vi "lbvproject.vi"() -> ()   [LabVIEW 2023]
uses:
  <vilib>/measure/mamon.llb/Waveform Peak Detection for N Chan.vi
  <vilib>/measure/NI_MAPro.lvlib
panel:
  out "Histogram":dynamicdata(graph)
  out "windowed monitor (post filter)":dynamicdata(graph)
  out "monitor chart":dynamicdata(graph)
  in  "stop":bool
  out "heart rate (bpm)":dbl
  out "frequency in Hz":dbl
  out "Scalar":dbl
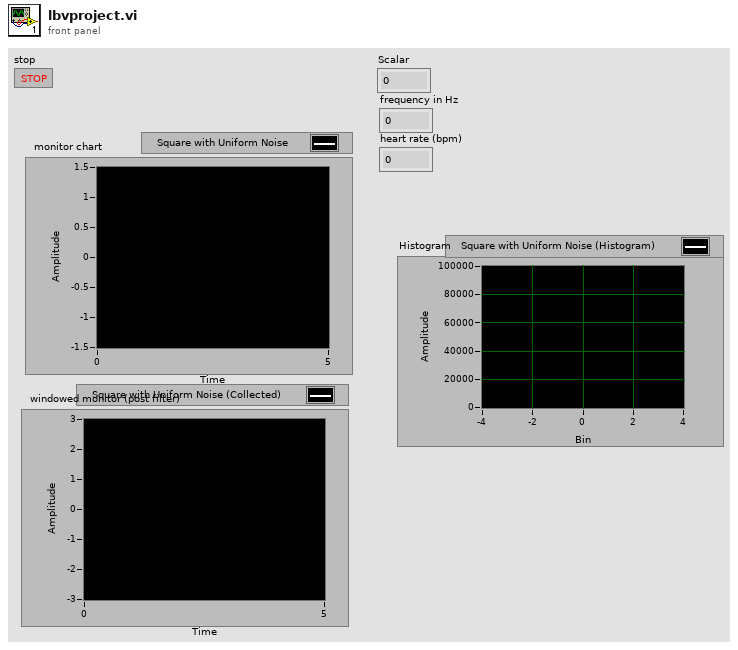
[diagram p1: front panel]
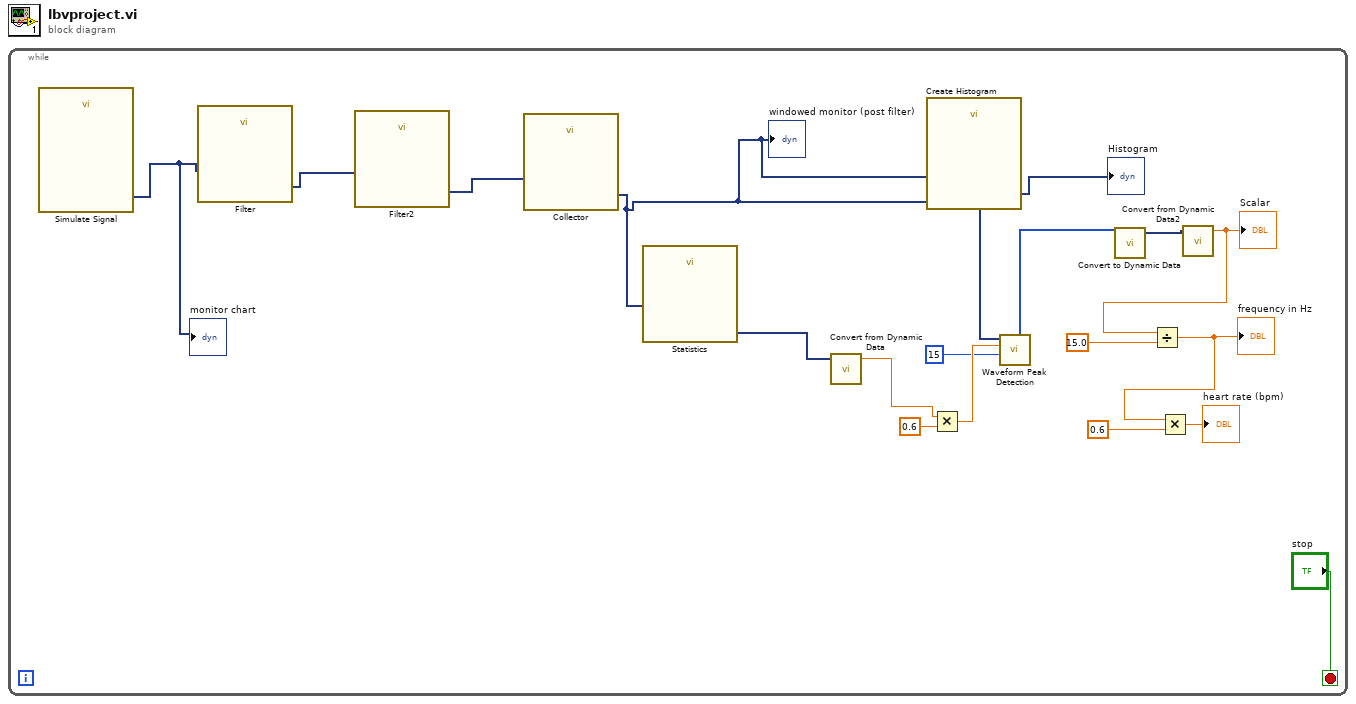
[diagram p0: block diagram]
diagram:
  n1 = while {
    stop <- "stop" stop-if-true
    n2 = call "Simulate Signal"() -> ("Square with Uniform Noise"=w3:dynamicdata)  [unwired: 14 in, 1 out]
    "monitor chart" <- w3
    n3 = call "Filter"("Signal"=w3) -> ("Filtered Signal"=w18:dynamicdata)  [unwired: 9 in, 1 out]
    n4 = call "Filter2"("Signal"=w18) -> ("Filtered Signal"=w17:dynamicdata)  [unwired: 9 in, 1 out]
    n5 = call "Collector"("Signals"=w17) -> ("Collected Signals"=w1:dynamicdata)  [unwired: 9 in, 1 out]
    "windowed monitor (post filter)" <- w1
    n6 = call "Statistics"("Signals"=w1) -> ("Maximum"=w16:dynamicdata)  [unwired: 25 in, 1 out]
    n7 = call "Convert from Dynamic Data"("Dynamic Data Type"=w16) -> ("Scalar"=w14:dbl)  [unwired: 3 in]
    n8 = call "Create Histogram"("Signal"=w1) -> ("Histogram"=→"Histogram":dynamicdata)  [unwired: 9 in, 1 out]
    n9 = Multiply(x=w14, y=0.6) -> (x*y=w13:dbl)
    n10 = call-poly <vilib>:"Waveform Peak Detection.vi"("width"=15, "threshold"=w13, "Signals In"=w1) -> ("# found"=w11:i32[])  [unwired: 4 in, 4 out]
    n11 = call "Convert to Dynamic Data"("Array"=w11) -> ("Dynamic Data Type"=w10:dynamicdata)  [unwired: 3 in]
    n12 = call "Convert from Dynamic Data2"("Dynamic Data Type"=w10) -> ("Scalar"=w9:dbl)  [unwired: 3 in]
    "Scalar" <- w9
    n13 = Divide(x=w9, y=15.0) -> (x/y=w7:dbl)
    "frequency in Hz" <- w7
    n14 = Multiply(x=w7, y=0.6) -> (x*y=→"heart rate (bpm)":dbl)
  }
